vi "Get Supported Targets.vi"(8 "error in":errorcluster, 11 "TDMS datalogger configuration in":refnum<class "TDMS datalogger configuration.lvclass">) -> (0 "error out":errorcluster, 2 "supported targets":T1[](array[typedef]), 3 "TDMS datalogger configuration out":refnum<class "TDMS datalogger configuration.lvclass">)   [LabVIEW 2013, in "TDMS datalogger configuration.lvclass"]
doc: "Provides an interface for determining the targets supported by a given module configuration/runtime class pairing. This should be overridden by any useful child class."
uses:
  TDMS datalogger configuration.lvclass
  <vilib>/NI/Tag Bus Module Framework/root configuration/Target Types.ctl
  <vilib>/NI/Tag Bus Module Framework/root configuration/TBM configuration.lvclass
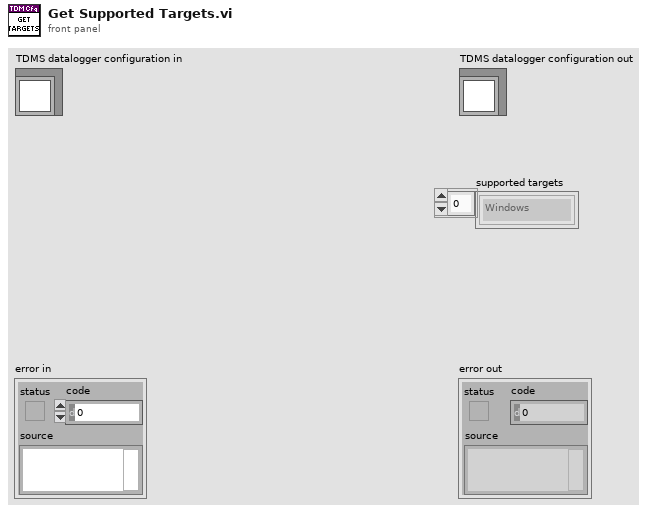
[diagram p1: front panel]
types:
  T1 = typedef "TBM configuration.lvclass/Target Types.ctl" = enum16{"Windows", "Mac", "Linux", "Linux RT", "VxWorks", "Pharlap", "Other"}
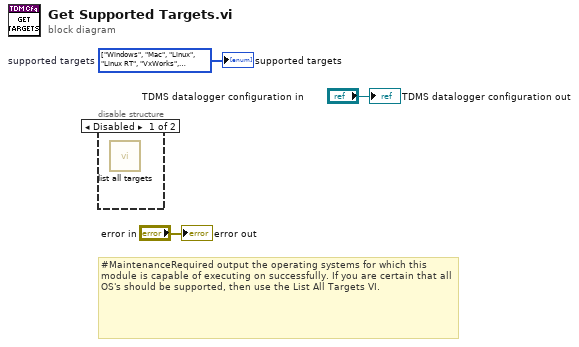
[diagram p0: block diagram]
diagram:
  w1 = T1[] [enum."Windows", enum."Mac", enum."Linux", enum."Linux RT", enum."VxWorks", enum."Pharlap"] items=["Windows", "Mac", "Linux", "Linux RT", "VxWorks", "Pharlap", "Other"]  # supported targets
  # "#MaintenanceRequired output the operating systems for which this module is capable of executing on successfully. If you are certain that all OS's should be supported, then use the List All Targets VI."
  n1 = disable-structure shown="Disabled" {
    frame Disabled {
      n2 = call <vilib>:"list all targets.vi"() -> ()  [unwired: 11 in, 1 out]
    }
    frame Enabled {
    }
  }
  "error out" <- "error in"
  "TDMS datalogger configuration out" <- "TDMS datalogger configuration in"
  "supported targets" <- w1
